vi "in_derivatives for Hermite.vi"(0 "Y[0..N]":dbl[](array[numeric]) format="%_6g", 1 "X[0..N]":dbl[](array[numeric]) format="%_6g") -> (7 "Y deriv[0..N]":dbl[](array[numeric]) format="%_6g")   [LabVIEW 2020, in "NI_Gmath.lvlib"]
uses:
  NI_Gmath.lvlib
panel:
  out "derivatives":cluster{"X[0..N]":dbl[], "Y[0..N]":dbl[]}[](graph)
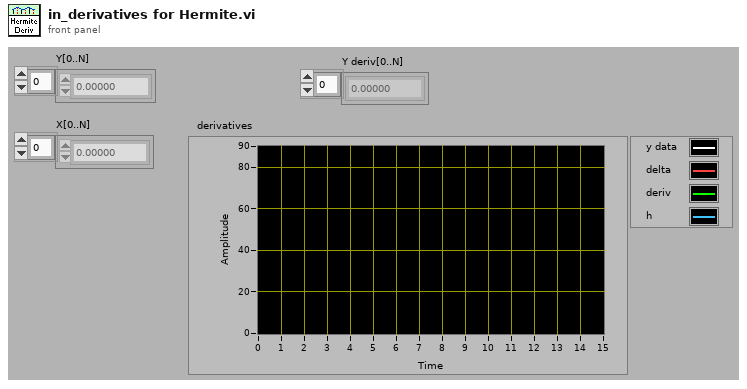
[diagram p1: front panel]
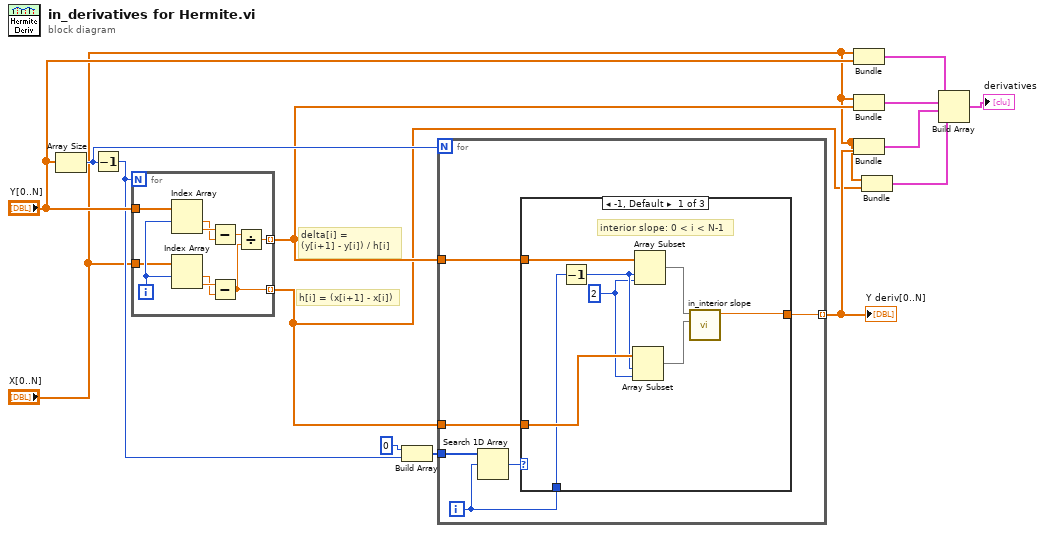
[diagram p0: block diagram]
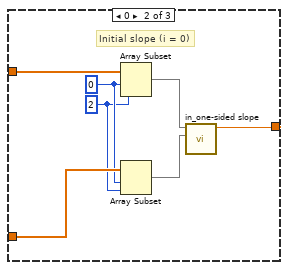
[diagram p2: hidden frame]
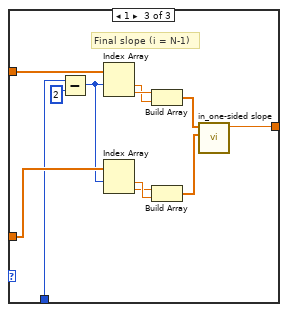
[diagram p3: hidden frame]
diagram:
  # "delta[i] =\n(y[i+1] - y[i]) / h[i]"
  # "h[i] = (x[i+1] - x[i])"
  n1 = Array Size(array="Y[0..N]") -> (size(s)=w14:i32)
  n2 = Decrement(x=w14) -> (x-1=w5:i32)
  n3 = for {
    N: w5 -> [_]
    tunnel: "Y[0..N]" -> [w24]
    tunnel: [w20] -> w6 mode=indexing
    tunnel: "X[0..N]" -> [w16]
    tunnel: [w15] -> w2 mode=indexing
    i -> [w19]
    n4 = Index Array(array=w24, index #1=w19) -> (element #1=w22:dbl, element #2=w23:dbl)  [unwired: 1 in]
    n5 = Index Array(array=w16, index #1=w19) -> (element #1=w17:dbl, element #2=w18:dbl)  [unwired: 1 in]
    n6 = Subtract(x=w23, y=w22) -> (x-y=w21:dbl)
    n7 = Subtract(x=w18, y=w17) -> (x-y=w15:dbl)
    n8 = Divide(x=w21, y=w15) -> (x/y=w20:dbl)
  }
  n9 = Build Array(0 ("element"), w5) -> (w12:i32[])
  n10 = for {
    N: w14 -> [_]
    tunnel: [w30] -> w10 mode=indexing
    tunnel: w2 -> [w28]
    tunnel: w6 -> [w27]
    tunnel: w12 -> [w26]
    i -> [w25]
    n11 = Search 1D Array(1D array=w26, element=w25) -> (index of element=w29:i32)  [unwired: 1 in]
    n12 = case shown="-1, Default" w29 {
      tunnel: [w36 w43 w56] -> w30
      tunnel: w28 -> [w37 w44 w55]
      tunnel: w27 -> [w38 w45 w57]
      tunnel: w25 -> [w34 _ w48]
      frame -1, Default {
        w31 = 2 ("index")
        # "interior slope: 0 < i < N-1"
        n13 = Decrement(x=w34) -> (x-1=w35:i32)
        n14 = Array Subset(array=w37, index=w35, length=w31) -> (w32:dbl[])
        n15 = Array Subset(array=w38, index=w35, length=w31) -> (w33:dbl[])
        n16 = call "in_interior slope.vi"("h[0..1]"=w32, "delta[0..1]"=w33) -> ("interior slope"=w36:dbl)  [unwired: 9 in]
      }
      frame 0 {
        w41 = 2 ("index")
        w42 = 0 ("index")
        # "Initial slope (i = 0)"
        n17 = Array Subset(array=w45, index=w42, length=w41) -> (w40:dbl[])
        n18 = Array Subset(array=w44, index=w42, length=w41) -> (w39:dbl[])
        n19 = call "in_one-sided slope.vi"("h[0..1]"=w39, "delta[0..1]"=w40) -> ("one-sided slope"=w43:dbl)  [unwired: 9 in]
      }
      frame 1 {
        # "Final slope (i = N-1)"
        n20 = Subtract(x=w48, y=2) -> (x-y=w46:i32)
        n21 = Index Array(array=w57, index #1=w46) -> (element #1=w51:dbl, element #2=w52:dbl)  [unwired: 1 in]
        n22 = Index Array(array=w55, index #1=w46) -> (element #1=w54:dbl, element #2=w53:dbl)  [unwired: 1 in]
        n23 = Build Array(w52, w51) -> (w50:dbl[])
        n24 = Build Array(w53, w54) -> (w49:dbl[])
        n25 = call "in_one-sided slope.vi"("h[0..1]"=w49, "delta[0..1]"=w50) -> ("one-sided slope"=w56:dbl)  [unwired: 9 in]
      }
    }
  }
  "Y deriv[0..N]" <- w10
  n26 = Bundle("X[0..N]"="X[0..N]", "Y[0..N]"="Y[0..N]") -> (w9:cluster{"X[0..N]":dbl[], "Y[0..N]":dbl[]})  [unwired: 1 in]
  n27 = Bundle("X[0..N]"="X[0..N]", w6) -> (w8:cluster{"X[0..N]":dbl[], dbl[]})  [unwired: 1 in]
  n28 = Bundle("X[0..N]"="X[0..N]", w10) -> (w4:cluster{"X[0..N]":dbl[], dbl[]})  [unwired: 1 in]
  n29 = Bundle("X[0..N]"="X[0..N]", w2) -> (w1:cluster{"X[0..N]":dbl[], dbl[]})  [unwired: 1 in]
  n30 = Build Array(w9, w8, w4, w1) -> (→"derivatives":cluster{"X[0..N]":dbl[], "Y[0..N]":dbl[]}[])
